vi "setUp.vi"(8 "error in (no error)":errorcluster, 11 "reference in":refnum<class "Routing and Faulting Export Unit Tests.lvclass">) -> (0 "error out":errorcluster, 3 "reference out":refnum<class "Routing and Faulting Export Unit Tests.lvclass">)   [LabVIEW 2020, in "Routing and Faulting Export Unit Tests.lvclass"]
doc: "setUp runs prior to the test method during test execution. Use this method to initialize any object data required by your tests."
uses:
  Routing and Faulting Export Unit Tests.lvclass
  C:/Program Files (x86)/National Instruments/LabVIEW 2020/vi.lib/addons/_JKI Toolkits/VI Tester/TestCase.llb/TestCase.lvclass
  NationalInstruments.VeriStand.SystemDefinitionAPI
  Routing and Faulting Export Unit Tests.lvclass/Routing and Faulting Export Unit Tests.ctl
  <userlib>/_OpenG.lib/file/file.llb/Append Path to Root if Relative - Scalar__ogtk.vi
  <vilib>/addons/_JKI Toolkits/VI Tester/TestCase.llb/TestCase.lvclass
  niveristand-custom-device-testing-tools/VeriStandTestUtilities/VeriStandTestUtilities.lvlib
  Scripting/Routing and Faulting Scripting.lvlib
  <vilib>/NI/NI VeriStand Custom Device Import and Export Tool/ImportExport.lvlib
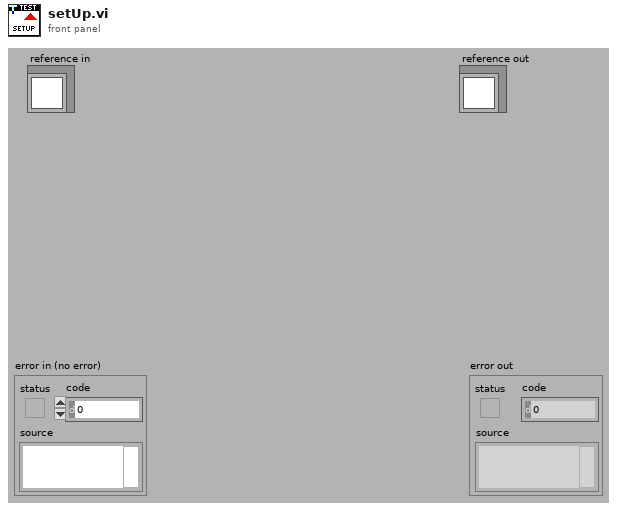
[diagram p1: front panel]
types:
  T1 = typedef "Custom Device API.lvlib/Custom Device Item Ref.ctl" = u64
  T2 = typedef "Advanced System Definition.lvlib/SysDef.Export.ctl" = cluster{"Version":string, "Tree":T3[]}
  T3 = typedef "Advanced System Definition.lvlib/TreeItem.ctl" = cluster{"Item Info":T4, "Parent Path":string[], "Properties":T9[]}
  T4 = typedef "Advanced System Definition.lvlib/TreeItem.Info.ctl" = cluster{"Name":string, "Description":string, "GUID":string, "Is Channel":bool, "Channel":T5, "Is Waveform":bool, "Waveform":T7}
  T5 = typedef "Custom Device API.lvlib/Custom Device Channel.ctl" = cluster{"Type":T6, "Units":string, "Default Value":dbl, "Faultable":bool, "Scalable":bool}
  T6 = typedef "Custom Device API.lvlib/Custom Device Channel Type.ctl" = enum16{"Input", "Output"}
  T7 = typedef "Custom Device API.lvlib/Custom Device Waveform.ctl" = cluster{"Data Type":T8, "Units":string}
  T8 = typedef "Custom Device API.lvlib/Custom Device Waveform DataType.ctl" = enum16{"Double", "Complex Double"}
  T9 = typedef "Advanced System Definition.lvlib/TreeItem.Property.ctl" = cluster{"Name":string, "Type":i32, "Value":variant}
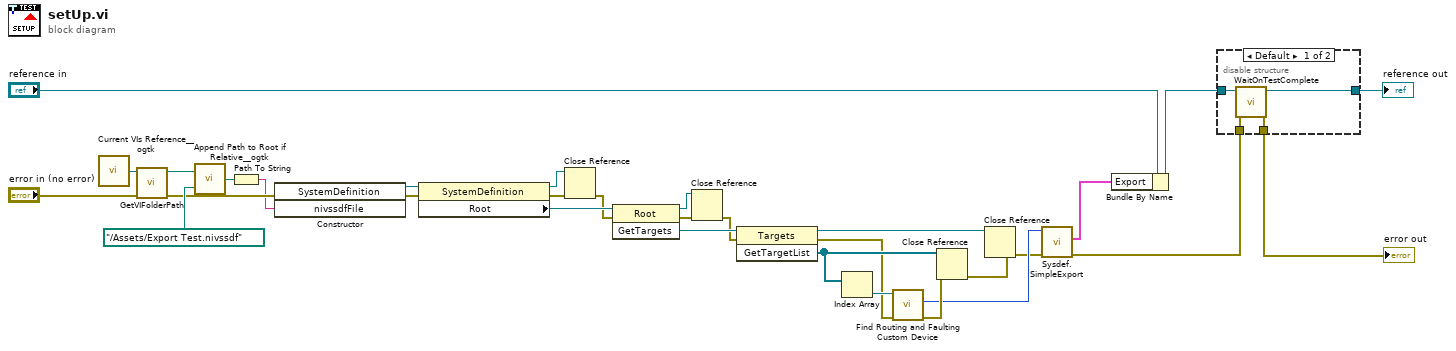
[diagram p0: block diagram]
diagram:
  n1 = call <userlib>:"Current VIs Reference__ogtk.vi"() -> ("Current VI's reference"=w27:refnum<vi>)  [unwired: 5 in]
  n2 = call "GetVIFolderPath.vi"("error in (no error)"="error in (no error)", "VI Reference in"=w27) -> ("error out"=w23:errorcluster, "VI Folder Path out"=w26:path)  [unwired: 8 in]
  n3 = call-poly <userlib>:"Append Path to Root if Relative__ogtk.vi"("Absolute or Relative Path"=path "../Assets/Export Test.nivssdf", "Root Path"=w26) -> ("Absolute or Appended Path"=w24:path)
  n4 = Path To String(path=w24) -> (string=w21:string)
  n5 = constructor class="SystemDefinition"(error in=w23, "nivssdfFile"=w21) -> (reference out=w20:refnum<k24>, error out=w22:errorcluster)  [unwired: 2 in, 2 out]
  n6 = property class="SystemDefinition"(reference=w20, error in=w22) -> (reference out=w13:refnum<k24>, error out=w15:errorcluster, "Root"=w19:refnum<k24>)
  n7 = Close Reference(reference=w13, error in (no error)=w15) -> (error out=w14:errorcluster)
  n8 = invoke class="Root" method="GetTargets"(reference=w19, error in=w14) -> (reference out=w10:refnum<k24>, error out=w12:errorcluster, "GetTargets"=w18:refnum<k24>)  [unwired: 1 in]
  n9 = Close Reference(reference=w10, error in (no error)=w12) -> (error out=w11:errorcluster)
  n10 = invoke class="Targets" method="GetTargetList"(reference=w18, error in=w11) -> (reference out=w16:refnum<k24>, error out=w4:errorcluster, "GetTargetList"=w9:refnum<k24>[])  [unwired: 1 in]
  n11 = Index Array(array=w9) -> (element=w8:refnum<k24>)  [unwired: 1 in]
  n12 = call "Find Routing and Faulting Custom Device.vi"("error in"=w4, "target in"=w8) -> ("error out"=w3:errorcluster, "routing and faulting custom device"=w2:T1)  [unwired: 7 in, 1 out]
  n13 = Close Reference(reference=w9, error in (no error)=w3) -> (error out=w17:errorcluster)
  n14 = Close Reference(reference=w16, error in (no error)=w17) -> (error out=w1:errorcluster)
  n15 = call <vilib>:"Sysdef.SimpleExport.vi"("error in (no error)"=w1, "ID"=w2) -> ("error out"=w6:errorcluster, "Export"=w5:T2)  [unwired: 7 in, 1 out]
  n16 = Bundle By Name(cluster="reference in", "Export"=w5) -> (w28:refnum<class "Routing and Faulting Export Unit Tests.lvclass">)
  n17 = disable-structure shown="Default" {
    disable-tunnel: w6 -> [w35 w36]
    disable-tunnel: [w34 w36] -> w31
    disable-tunnel: [w33 w37] -> w29
    disable-tunnel: w28 -> [w32 w37]
    frame condition #0 (active) {
      n18 = call <vilib>:"WaitOnTestComplete.vi"("error in (no error)"=w35, "TestCase in"=w32) -> ("error out"=w34:errorcluster, "TestCase out"=w33:refnum<class "Routing and Faulting Export Unit Tests.lvclass">)  [unwired: 8 in]
    }
    frame condition #1 {
    }
  }
  "error out" <- w31
  "reference out" <- w29
